vi "One or More Ignore Inputs.vi"(8 "error in (no error)":errorcluster, 11 "Mock in":refnum<class "Mock.lvclass">) -> (0 "error out":errorcluster, 3 "Mock out":refnum<class "Mock.lvclass">)   [LabVIEW 2020, in "One or More.lvlib"]
uses:
  One or More.lvlib
  Framework/Mock/Mock.lvclass
  Comparators/Any Inputs Comparator/Any Inputs Comparator.lvclass
  C:/git/astemes-lmock/source/Core/Comparator/Comparator.lvclass
  One or More.lvclass
  C:/git/astemes-lmock/source/Core/Expectation/Expectation.lvclass
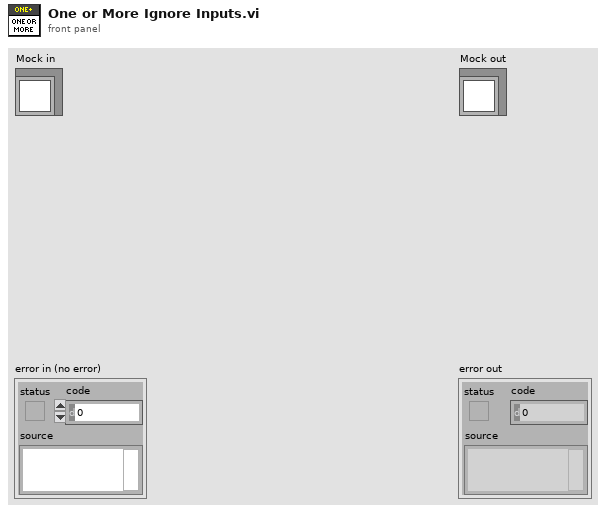
[diagram p1: front panel]
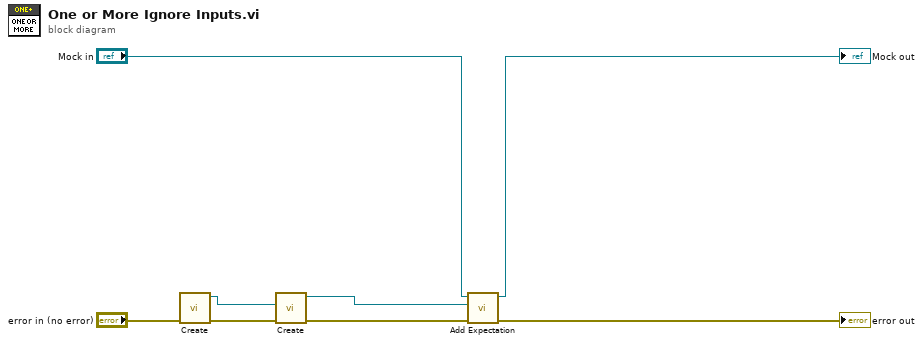
[diagram p0: block diagram]
diagram:
  n1 = call "Create.vi"("error in (no error)"="error in (no error)") -> ("error out"=w2:errorcluster, "Ignore Inputs Comparator"=w1:refnum<class "Any Inputs Comparator.lvclass">)  [unwired: 9 in]
  n2 = call "Create.vi"("error in (no error)"=w2, "Comparator"=w1) -> ("error out"=w4:errorcluster, "One or More"=w3:refnum<class "One or More.lvclass">)  [unwired: 8 in]
  n3 = call-dynamic "Add Expectation.vi"("error in (no error)"=w4, "Expectations"=w3, "Mock in"="Mock in") -> ("error out"=→"error out":errorcluster, "Mock out"=→"Mock out":refnum<class "Mock.lvclass">)  [unwired: 7 in]
